vi "Config - WriteFile.vi"(8 "Fehler (Eingang, kein Fehler)":errorcluster, 10 "DestinationFileName":string, 11 "SourceFullFileName":string) -> (0 "Fehler (Ausgang)":errorcluster)   [LabVIEW 2016]
uses:
  eGateUtility.dll
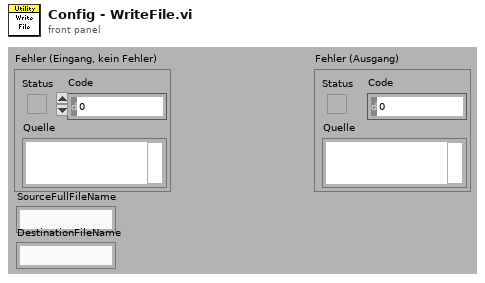
[diagram p1: front panel]
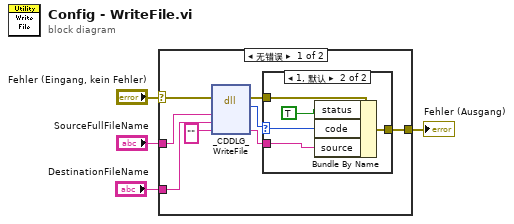
[diagram p0: block diagram]
diagram:
  n1 = case shown="无错误" "Fehler (Eingang, kein Fehler)" {
    selector: "Fehler (Eingang, kein Fehler)" -> [w12 w19]
    tunnel: [w10 w19] -> w3
    tunnel: "SourceFullFileName" -> [w6 _]
    tunnel: "DestinationFileName" -> [w5 _]
    frame No Error {
      n2 = dll-call lib="eGateUtility.dll" fn="_CDDLG_WriteFile"(error in=w12, "SourceFullFileName"=w6, "DestinationFileName"=w5, "ErrorString"="") -> (error out=w11:errorcluster, "Rückgabetyp"=w8:i32, "ErrorString"=w9:string)  [unwired: 4 in, 1 out]
      n3 = case shown="1, 默认" w8 {
        selector: w8 -> [_ w15]
        tunnel: w11 -> [w13 w18]
        tunnel: [w13 w17] -> w10
        tunnel: w9 -> [_ w16]
        frame 0 {
        }
        frame 1, Default {
          n4 = Bundle By Name(cluster=w18, "status"=TRUE, "code"=w15, "source"=w16) -> (w17:errorcluster)
        }
      }
    }
    frame Error {
    }
  }
  "Fehler (Ausgang)" <- w3
